vi "Read Waveform Measurement.vi"   [LabVIEW 2015, in "LeCroy Wave Series.lvlib"]
uses:
  <instrlib>/LeCroy Wave Series/LeCroy Wave Series.lvlib
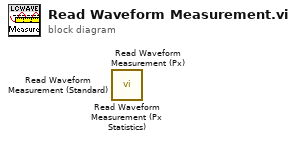
[diagram p0: block diagram]
diagram:
  n1 = call <instrlib>:"Read Waveform Measurement (Px Statistics).vi"() -> ()  [unwired: 6 in, 10 out]
  n2 = call <instrlib>:"Read Waveform Measurement (Px).vi"() -> ()  [unwired: 12 in, 4 out]
  n3 = call <instrlib>:"Read Waveform Measurement (Standard).vi"() -> ()  [unwired: 12 in, 4 out]
